vi "DynamicConfigData.OnCompile.Execute.vi"(8 "error in":errorcluster, 10 "VS Ref Groups":T2(array[cluster]) {"VS Refs" format="%.0x"}, 11 "Custom Device Ref":T1 format="%.0x") -> (0 "error out":errorcluster, 3 "Custom Device Ref":T1 format="%.0x")   [LabVIEW 2023, in "Data Access System Explorer.lvlib"]
uses:
  Data Access System Explorer.lvlib
  <vilib>/NI VeriStand/Custom Device API/Custom Device Item Ref.ctl
  <vilib>/NI VeriStand/Custom Device API/Data Reference.ctl
  <vilib>/NI VeriStand/Custom Device API/Block Data Reference.ctl
  <vilib>/NI VeriStand/Custom Device API/Data Access Type.ctl
  <vilib>/NI VeriStand/Custom Device API/Custom Device API.lvlib
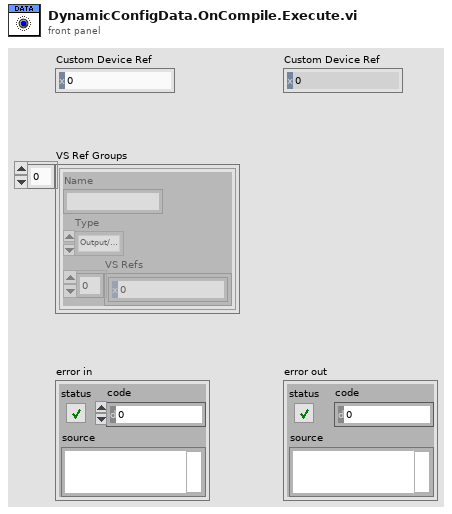
[diagram p1: front panel]
types:
  T1 = typedef "Custom Device API.lvlib/Custom Device Item Ref.ctl" = u64
  T2 = cluster{"Name":string, "Type":enum16{"Output/Write", "Input/Read", "Input/ReadWrite"}, "VS Refs":T1[]}[]
  T3 = typedef "Custom Device API.lvlib/Block Data Reference.ctl" = cluster{"Data Reference":T4, "Offset":u64, "Length":u64}
  T4 = typedef "Custom Device API.lvlib/Data Reference.ctl" = i32
  T5 = cluster{"Read":cluster{"Refs":T3[], "Values":dbl[]}[], "Write":cluster{"Refs":T3[], "Values":dbl[]}[], "ReadWrite":cluster{"Refs":T4[], "Values":dbl[], "Reset Values":dbl[]}[], "LUT":variant}
  T6 = cluster{"Refs":T4[], "Values":dbl[], "Reset Values":dbl[]}[]
  T7 = typedef "Custom Device API.lvlib/Data Access Type.ctl" = enum16{"Read", "Write"}
  T8 = cluster{"Refs":T4[], "Values":dbl[], "Reset Values":dbl[]}
  T9 = enum16{"Output/Write", "Input/Read", "Input/ReadWrite"}
  T10 = typedef "Custom Device API.lvlib/Custom Device Channel.ctl" = cluster{"Type":T11, "Units":string, "Default Value":dbl, "Faultable":bool, "Scalable":bool}
  T11 = typedef "Custom Device API.lvlib/Custom Device Channel Type.ctl" = enum16{"Input", "Output"}
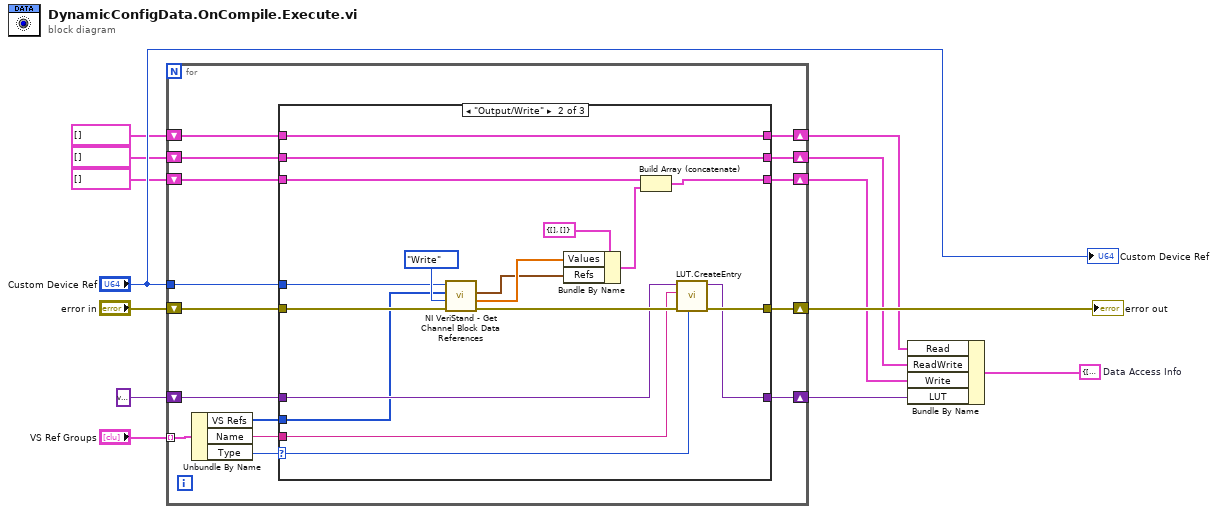
[diagram p0: block diagram]
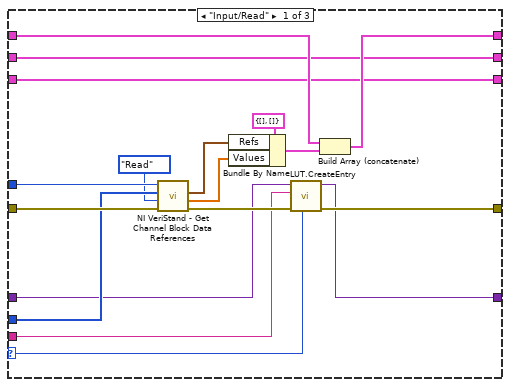
[diagram p2: hidden frame]
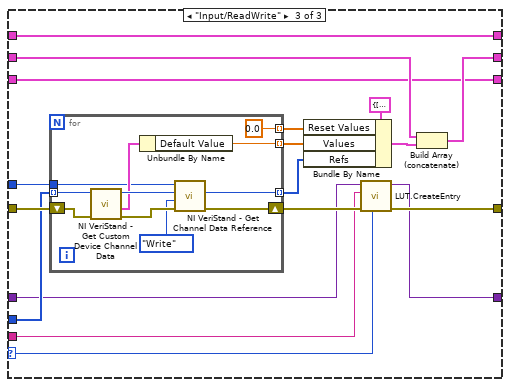
[diagram p3: hidden frame]
diagram:
  w10 = T5 {"Read"=[], "Write"=[], "ReadWrite"=[], "LUT"=variant}  # Data Access Info
  n1 = for {
    tunnel: "VS Ref Groups" -> [w26] mode=indexing
    shift-right: [w27] -> w12
    shift-left: "error in" -> [w28]
    tunnel: "Custom Device Ref" -> [w24]
    shift-right: [w22] -> w1
    shift-left: variant ("LUT") -> [w23]
    shift-right: [w21] -> w3
    shift-left: cluster{"Refs":T3[], "Values":dbl[]}[] [] -> [w16]
    shift-right: [w18] -> w2
    shift-left: T6 [] -> [w17]
    shift-right: [w15] -> w4
    shift-left: cluster{"Refs":T3[], "Values":dbl[]}[] [] -> [w14]
    n2 = Unbundle By Name(w26) -> ("VS Refs"=w25:T1[], "Name"=w20:string, "Type"=w19:T9)
    n3 = case shown="\"Output/Write\"" w19 {
      selector: w19 -> [w34 w58 w73]
      tunnel: w28 -> [w46 w63 w82]
      tunnel: [w45 w64 w80] -> w27
      tunnel: w25 -> [w43 w50 w75]
      tunnel: w24 -> [w42 w51 w70]
      tunnel: w23 -> [w41 w60 w72]
      tunnel: [w40 w59 w71] -> w22
      tunnel: [w31 w56 w65] -> w21
      tunnel: w20 -> [w35 w61 w74]
      tunnel: [w30 w57 w67] -> w18
      tunnel: w17 -> [w30 w57 w69]
      tunnel: w16 -> [w33 w56 w65]
      tunnel: [w29 w54 w66] -> w15
      tunnel: w14 -> [w29 w53 w66]
      frame "Input/Read" {
        n4 = call <vilib>:"NI VeriStand - Get Channel Block Data References.vi"("error in (no error)"=w46, "Access"=Data_Access_Type."Read", "Channel Refs"=w43, "Device Ref in"=w42) -> ("error out"=w44:errorcluster, "Values Array"=w37:dbl[], "Block Data Refs"=w38:T3[])  [unwired: 4 in, 1 out]
        n5 = Bundle By Name(cluster=cluster{"Refs":T3[], "Values":dbl[]} {"Refs"=[], "Values"=[]}, "Refs"=w38, "Values"=w37) -> (w32:cluster{"Refs":T3[], "Values":dbl[]})
        n6 = call "LUT.CreateEntry.vi"("Type"=w34, "error in (no error)"=w44, "Name"=w35, "LUT"=w41) -> ("error out"=w45:errorcluster, "LUT"=w40:variant)  [unwired: 6 in]
        n7 = Build Array (concatenate)(w33, w32) -> (w31:cluster{"Refs":T3[], "Values":dbl[]}[])
      }
      frame "Output/Write" {
        n8 = call <vilib>:"NI VeriStand - Get Channel Block Data References.vi"("error in (no error)"=w63, "Access"=Data_Access_Type."Write", "Channel Refs"=w50, "Device Ref in"=w51) -> ("error out"=w62:errorcluster, "Values Array"=w49:dbl[], "Block Data Refs"=w47:T3[])  [unwired: 4 in, 1 out]
        n9 = Bundle By Name(cluster=cluster{"Refs":T3[], "Values":dbl[]} {"Refs"=[], "Values"=[]}, "Values"=w49, "Refs"=w47) -> (w55:cluster{"Refs":T3[], "Values":dbl[]})
        n10 = Build Array (concatenate)(w53, w55) -> (w54:cluster{"Refs":T3[], "Values":dbl[]}[])
        n11 = call "LUT.CreateEntry.vi"("Type"=w58, "error in (no error)"=w62, "Name"=w61, "LUT"=w60) -> ("error out"=w64:errorcluster, "LUT"=w59:variant)  [unwired: 6 in]
      }
      frame "Input/ReadWrite" {
        n12 = for {
          shift-right: [w93] -> w81
          shift-left: w82 -> [w92]
          tunnel: [w87] -> w79 mode=indexing
          tunnel: [w86] -> w78 mode=indexing
          tunnel: [0.0] -> w77 mode=indexing
          tunnel: w75 -> [w84] mode=indexing
          tunnel: w70 -> [w83]
          n13 = call <vilib>:"NI VeriStand - Get Custom Device Channel Data.vi"("error in (no error)"=w92, "Channel Ref in"=w84) -> ("error out"=w91:errorcluster, "Channel"=w88:T10, "Channel Ref out"=w89:T1)  [unwired: 4 in, 3 out]
          n14 = Unbundle By Name(w88) -> ("Default Value"=w87:dbl)
          n15 = call <vilib>:"NI VeriStand - Get Channel Data Reference.vi"("error in (no error)"=w91, "Access"=Data_Access_Type."Write", "Channel Ref in"=w89, "Device Ref in"=w83) -> ("error out"=w93:errorcluster, "Channel Data Reference"=w86:T4)  [unwired: 5 in, 1 out]
        }
        n16 = Bundle By Name(cluster=T8 {"Refs"=[], "Values"=[], "Reset Values"=[]}, "Reset Values"=w77, "Values"=w79, "Refs"=w78) -> (w68:T8)
        n17 = call "LUT.CreateEntry.vi"("Type"=w73, "error in (no error)"=w81, "Name"=w74, "LUT"=w72) -> ("error out"=w80:errorcluster, "LUT"=w71:variant)  [unwired: 6 in]
        n18 = Build Array (concatenate)(w69, w68) -> (w67:T6)
      }
    }
  }
  "error out" <- w12
  n19 = Bundle By Name(cluster=w10, "Read"=w3, "ReadWrite"=w2, "Write"=w4, "LUT"=w1) -> ()  [unwired: 1 out]
  "Custom Device Ref" <- "Custom Device Ref"
